vi "CSM Batch Format Tool.vi"() -> ()   [LabVIEW 2017]
uses:
  _csmHelper/Utility/CSM Module Type.ctl
  <vilib>/Utility/miscctls.llb/LVRectTypeDef.ctl
  _csmHelper/API/Destroy.vi
  _csmHelper/API/Save Instrument.vi
  _csmHelper/API/Create From Basic Refs.vi
  _csmHelper/Utility/Is CSM Module - VIRef.vi
  _Shared/CSM Shared.lvlib
  _csmDoc/csmdoc.lvlib
  Communicable State Machine.lvlib
  _csmHelper/Utility/CSM-Helper Utility.lvlib
  _csmHelper/CSM-Helper.lvclass
  _csmHelper/API/Open Front Panel.vi
panel:
  in  "Enum":enum16{"Debugging", "AutoErrorHandling"}(ring)
  in  "Option":bool
  in  "Open":bool
  in  "CSM Only?":bool
  in  "Terminate":bool
  in  "Refresh":bool
  in  "Action: Update Connect Panel Doc":bool
  in  "Action: Set Debugging":bool
  in  "Macro: Open If Inline":bool
  in  "Macro: Update VI Title":bool
  in  "Macro: Relocate VI Window":bool
  in  "Macro: Rename Year of copyright":bool
  out "Listbox":i32(listbox)
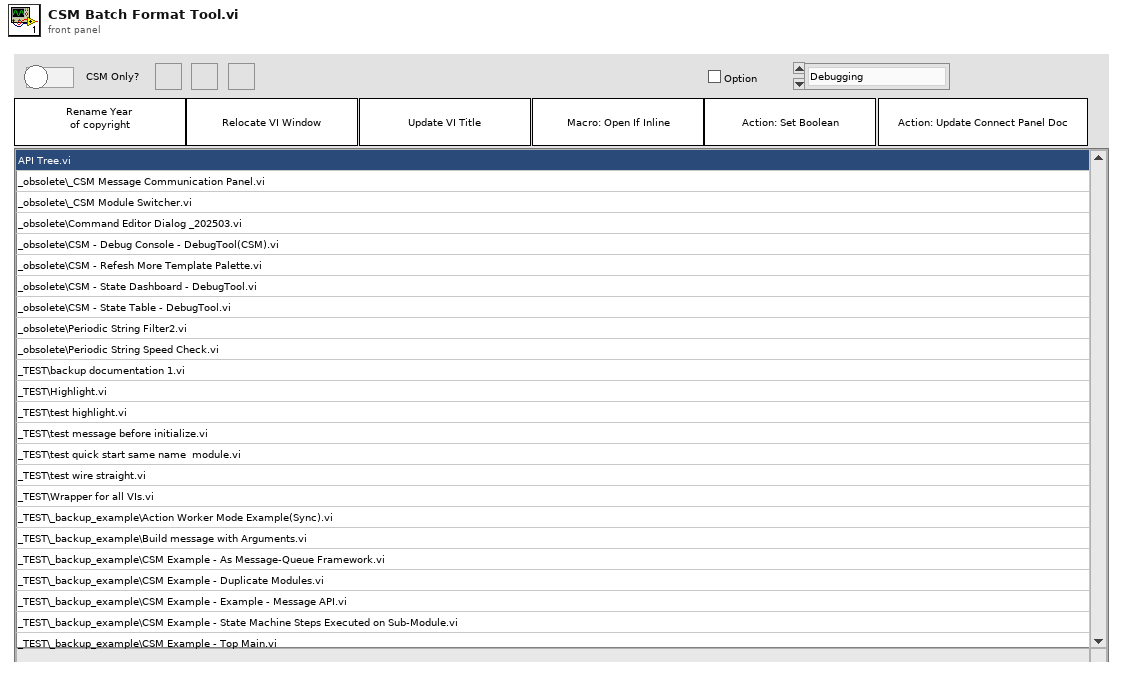
[diagram p1: front panel]
types:
  T1 = enum32{"Invalid", "Standard", "Closed", "Hidden", "Minimized", "Maximized"}
  T2 = enum32{"invalid app kind", "Development System", "Run Time System", "Student Edition", "Embedded LabVIEW", "Evaluation", "Custom"}
  T3 = typedef "CSM-Helper Utility.lvlib/CSM Module Type.ctl" = enum16{"Not a CSM", "JKISM", "CSM"}
  T4 = cluster{"Core":cluster{"Current VI Reference":refnum<vi>, "Close Panel on Exit?":bool}, "VIs":path[], "Success":bool, "Root":path}
  T5 = cluster{"Current VI Reference":refnum<vi>, "Close Panel on Exit?":bool}
  T6 = typedef "CSM-Helper Utility.lvlib/CSM Basic Refs.ctl" = cluster{"VI":refnum<vi>, "While Loop":refnum<vi>, "Case Structure":refnum<vi>, "Parse State Queue":refnum<vi>, "Event Structure":refnum<vi>, "Type":T3, "InLvlibp":bool}
  T7 = typedef "LVRectTypeDef.ctl" = cluster{"Left":i16, "Top":i16, "Right":i16, "Bottom":i16}
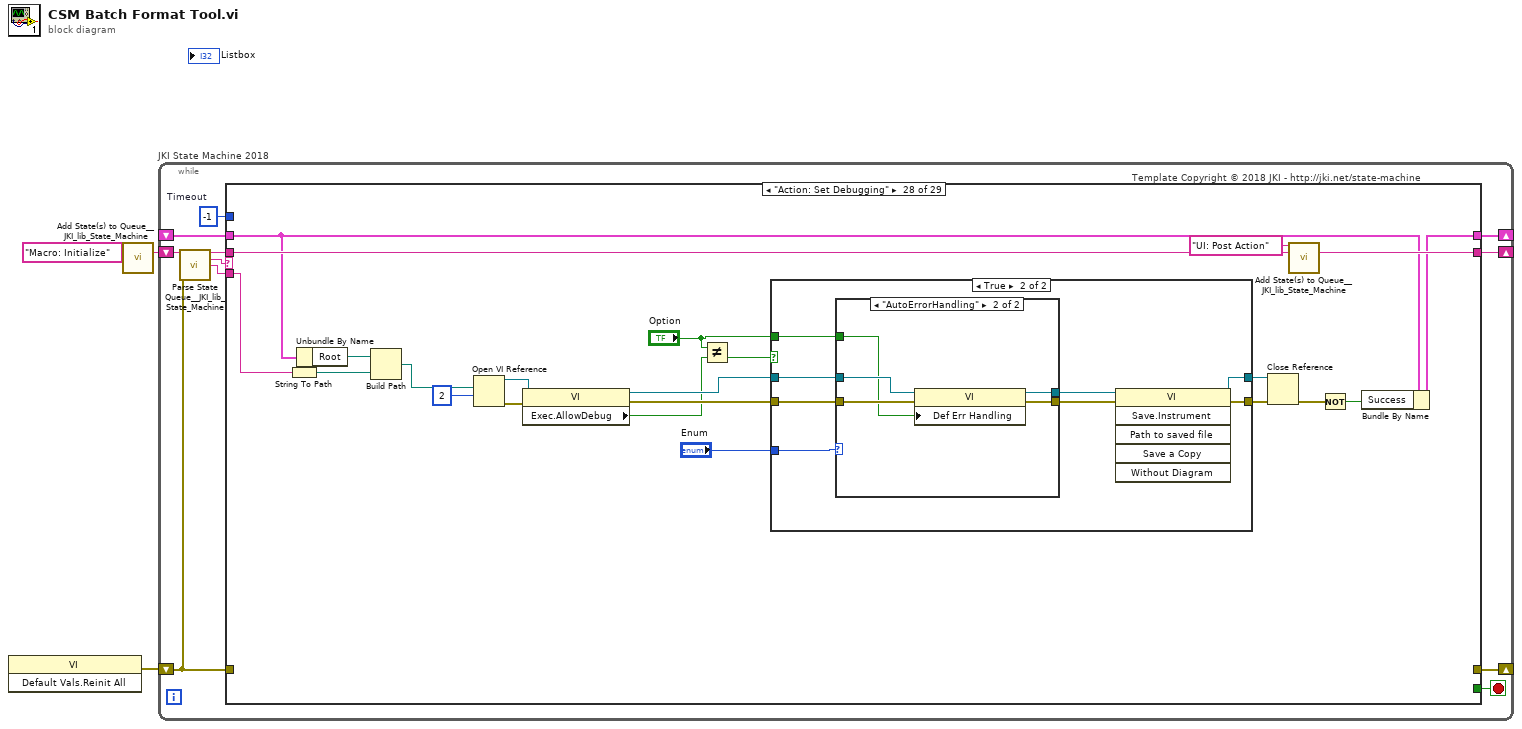
[diagram p0: block diagram]
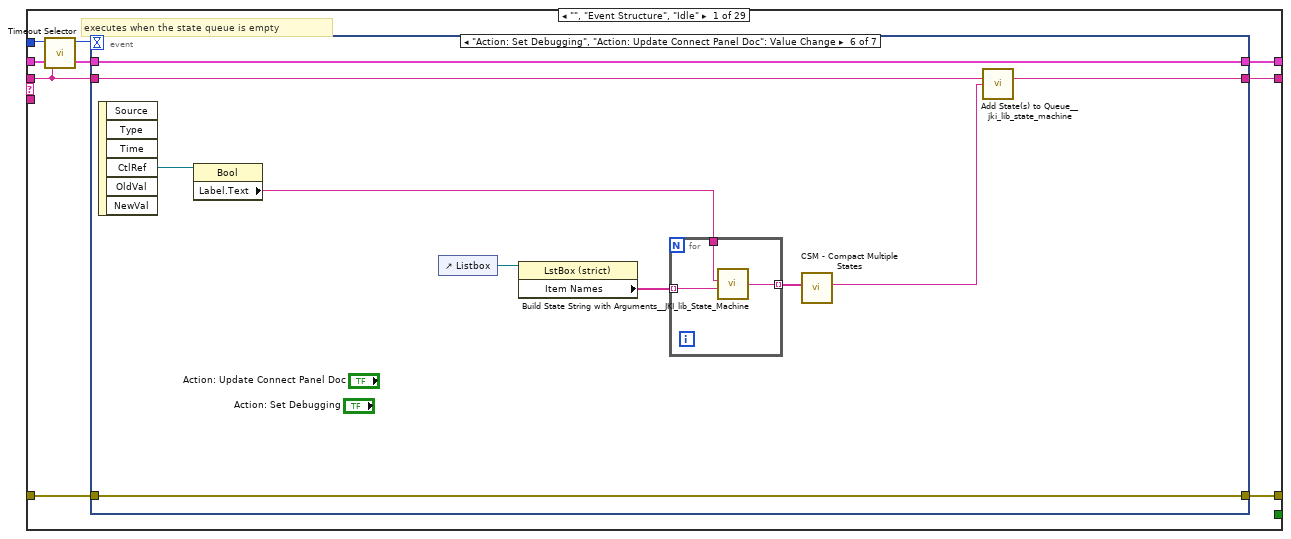
[diagram p2: hidden frame]
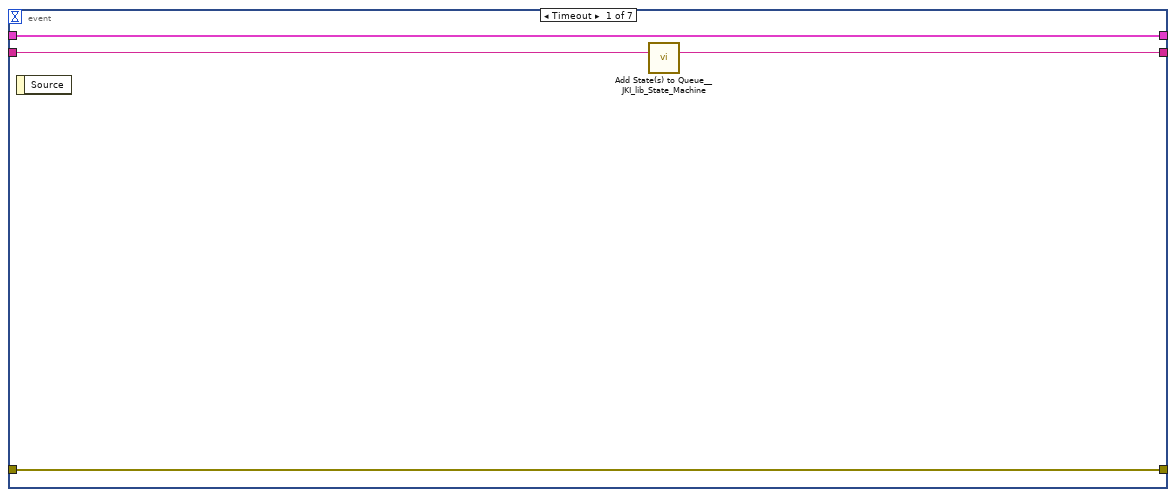
[diagram p3: hidden frame]
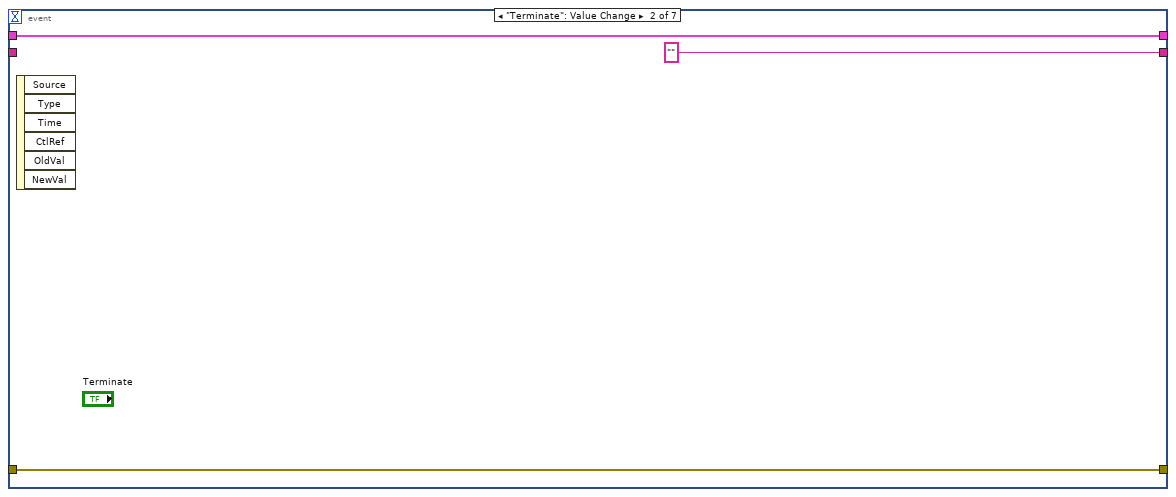
[diagram p4: hidden frame]
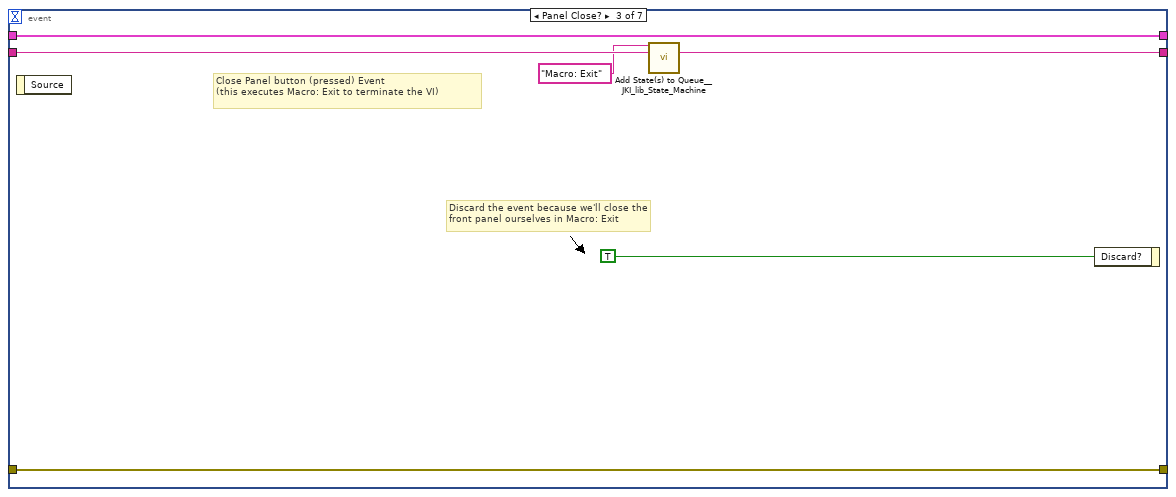
[diagram p5: hidden frame]
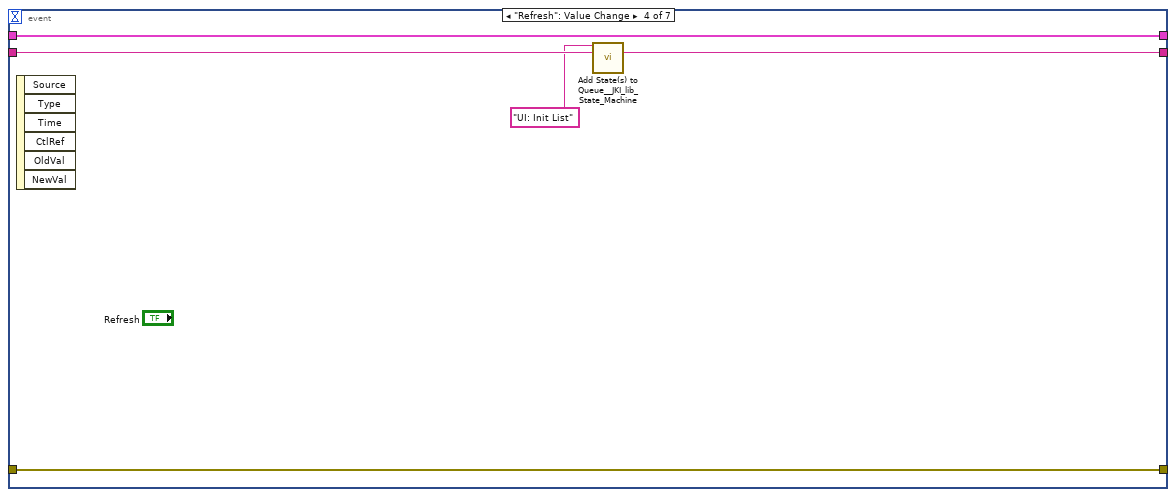
[diagram p6: hidden frame]
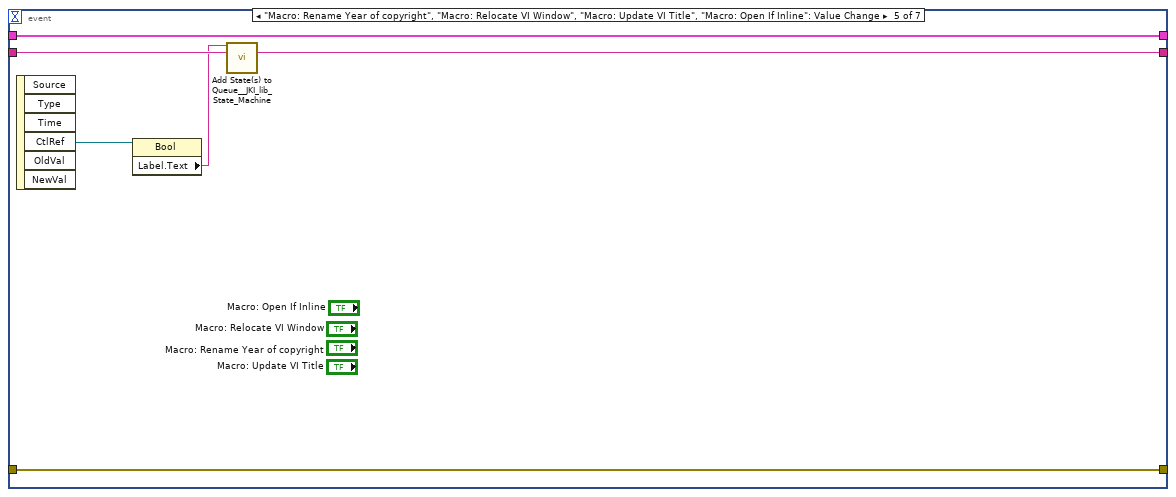
[diagram p7: hidden frame]
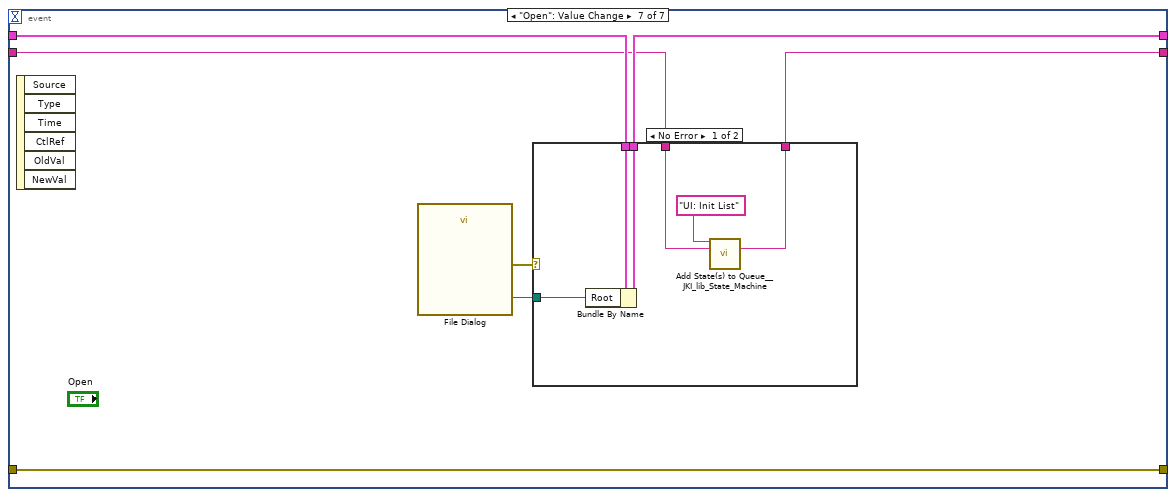
[diagram p8: hidden frame]
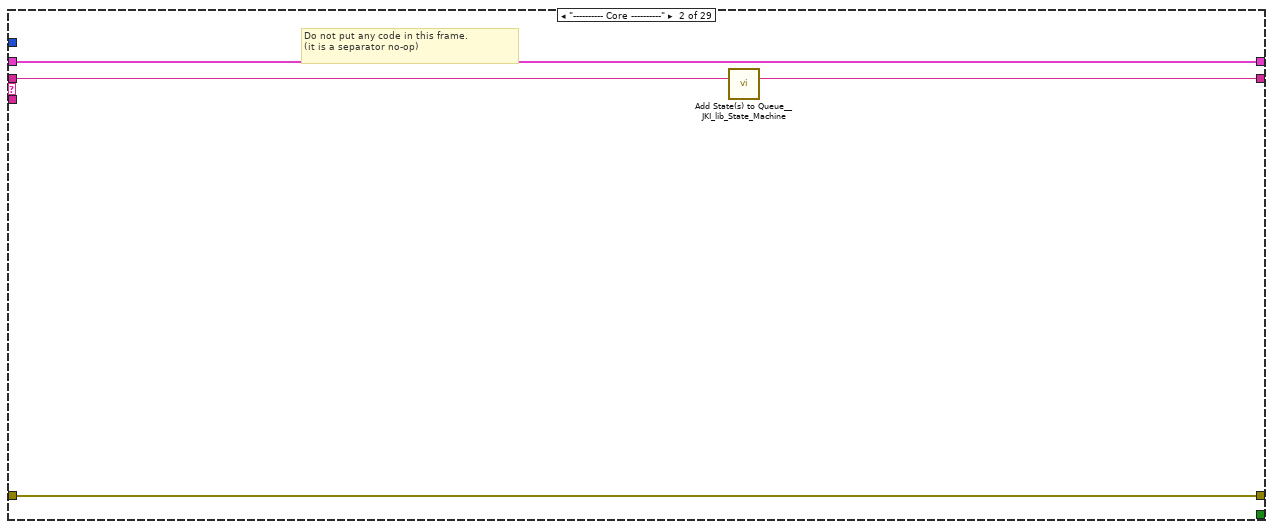
[diagram p10: hidden frame]
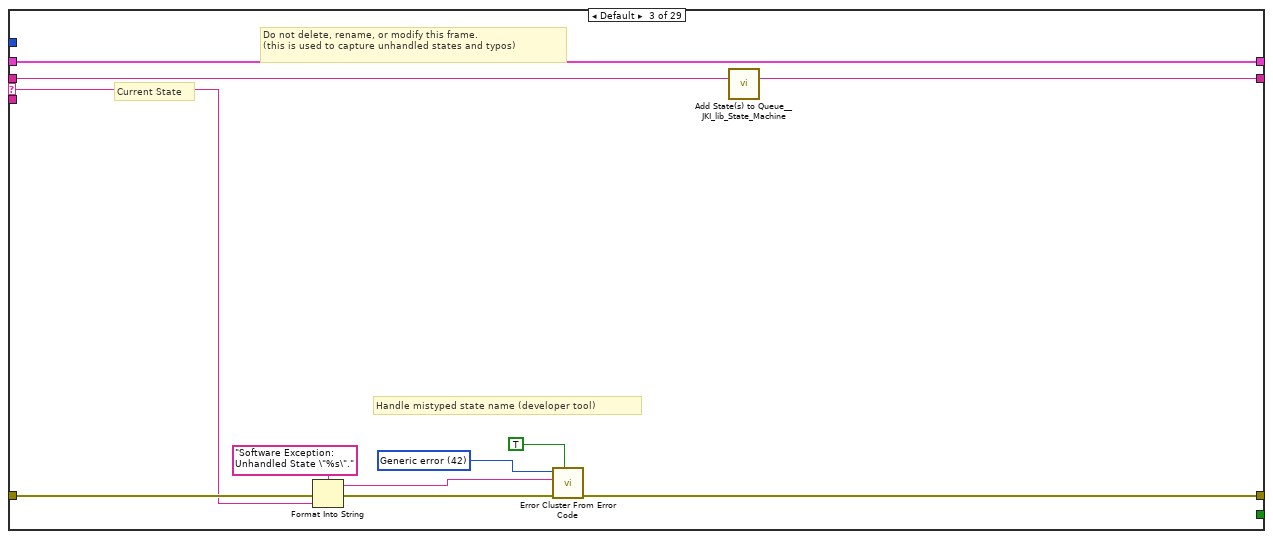
[diagram p11: hidden frame]
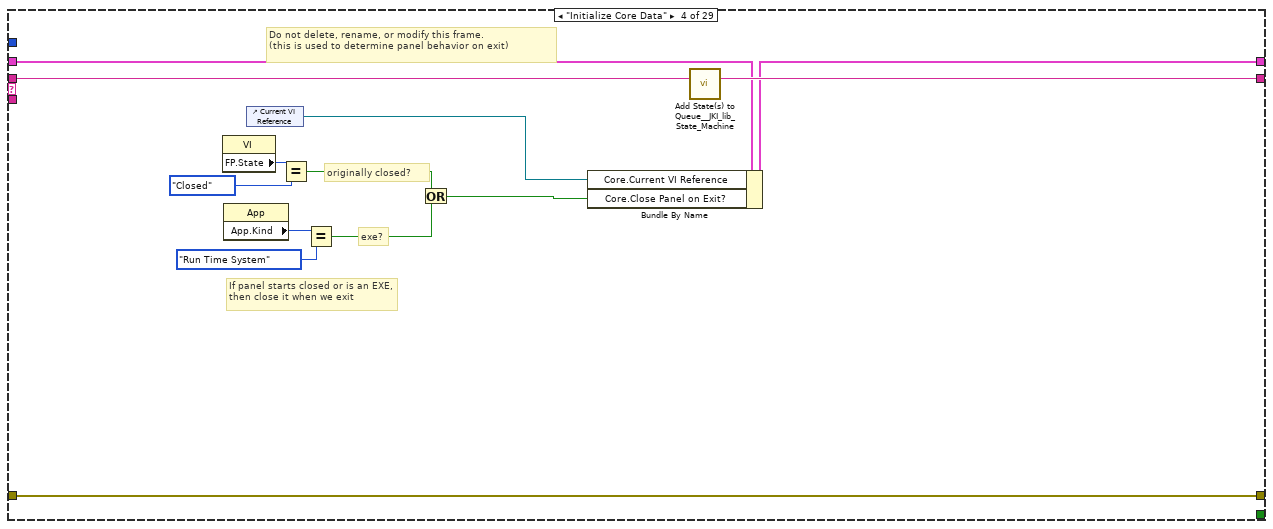
[diagram p12: hidden frame]
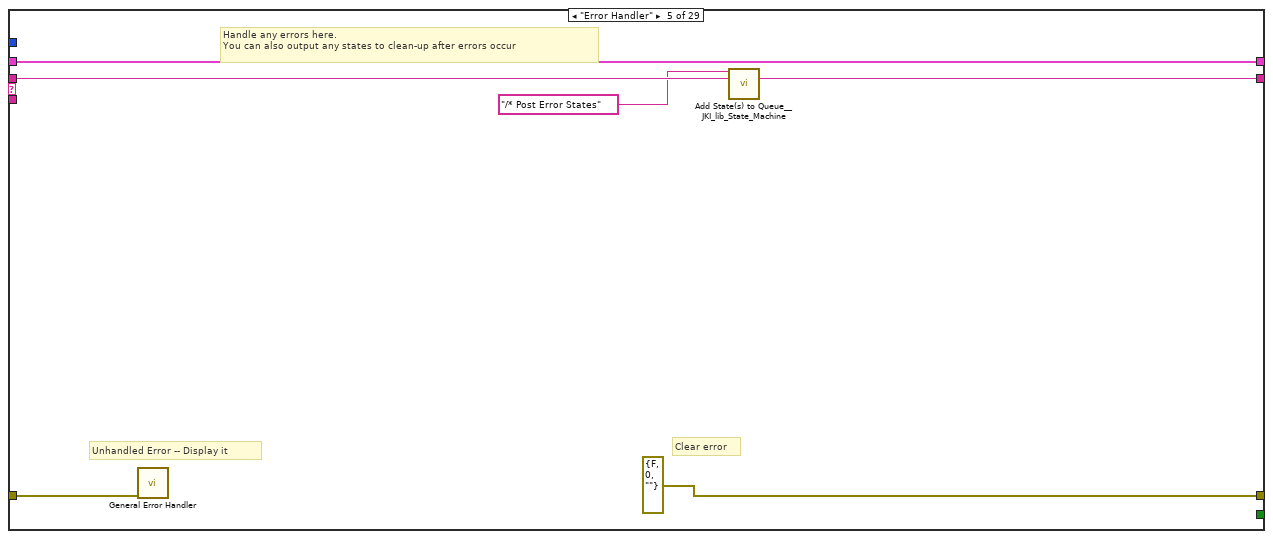
[diagram p13: hidden frame]
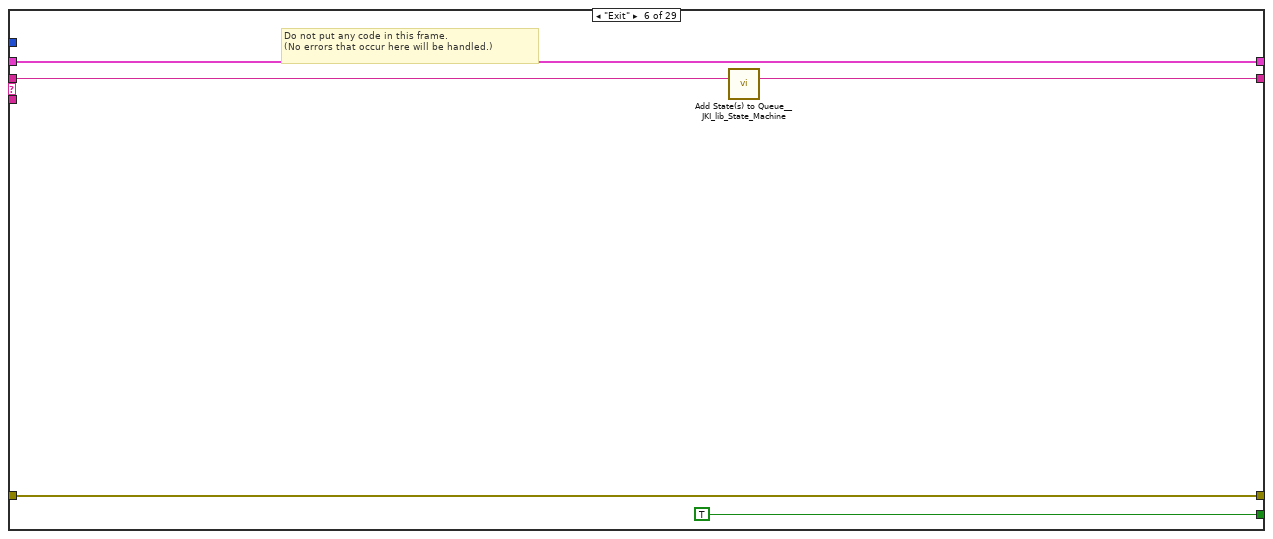
[diagram p14: hidden frame]
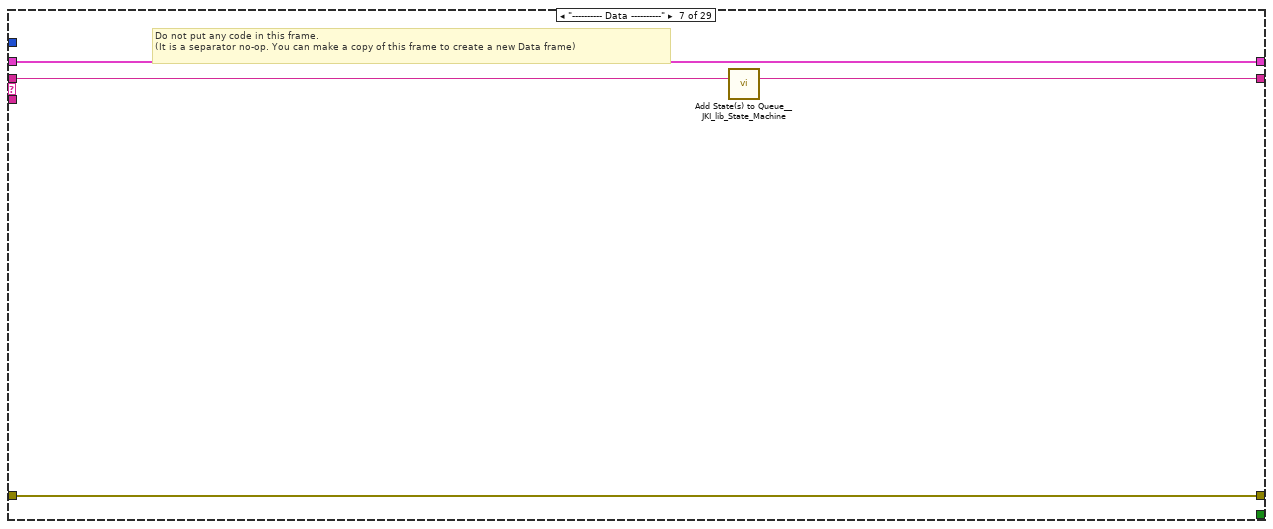
[diagram p15: hidden frame]
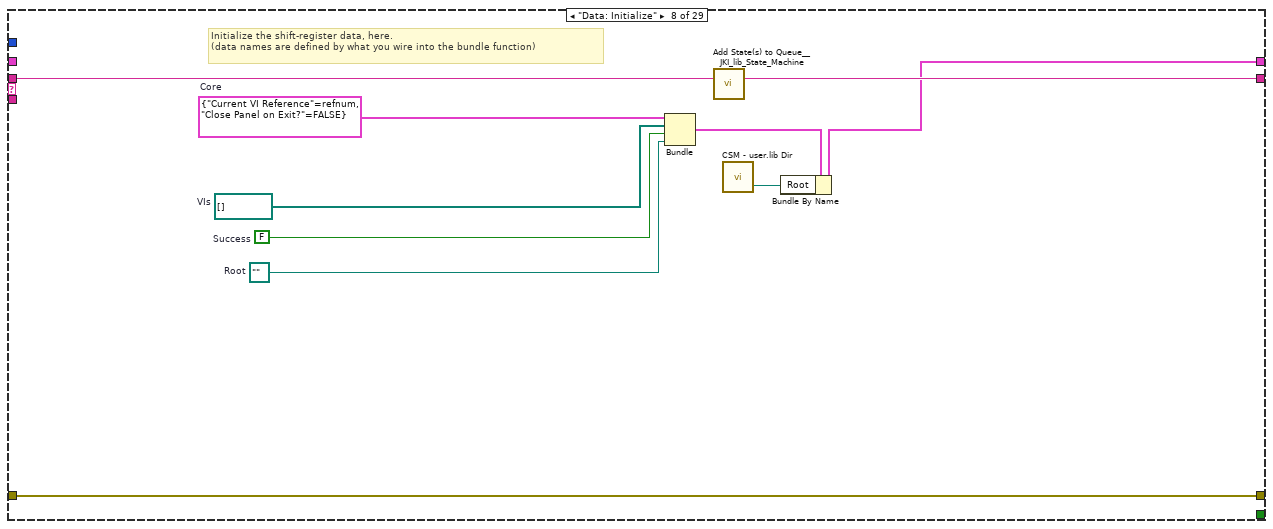
[diagram p16: hidden frame]
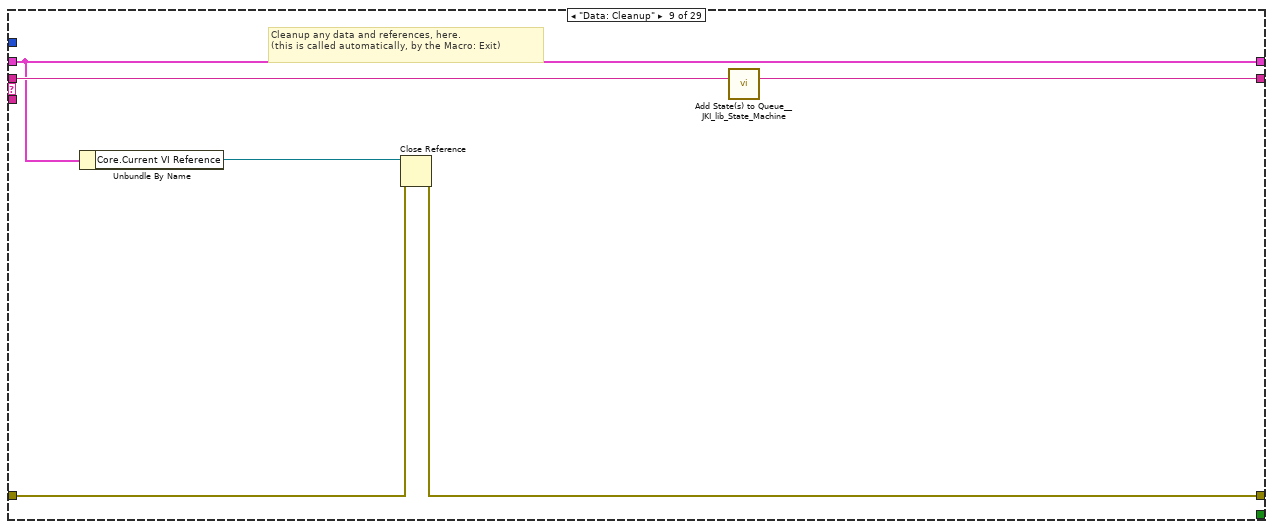
[diagram p17: hidden frame]
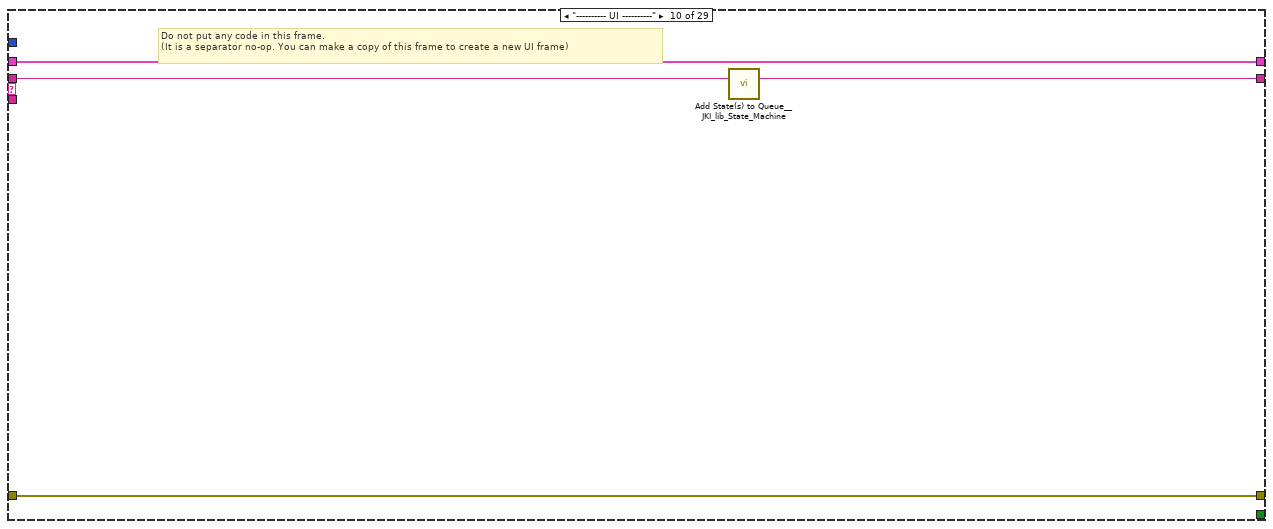
[diagram p18: hidden frame]
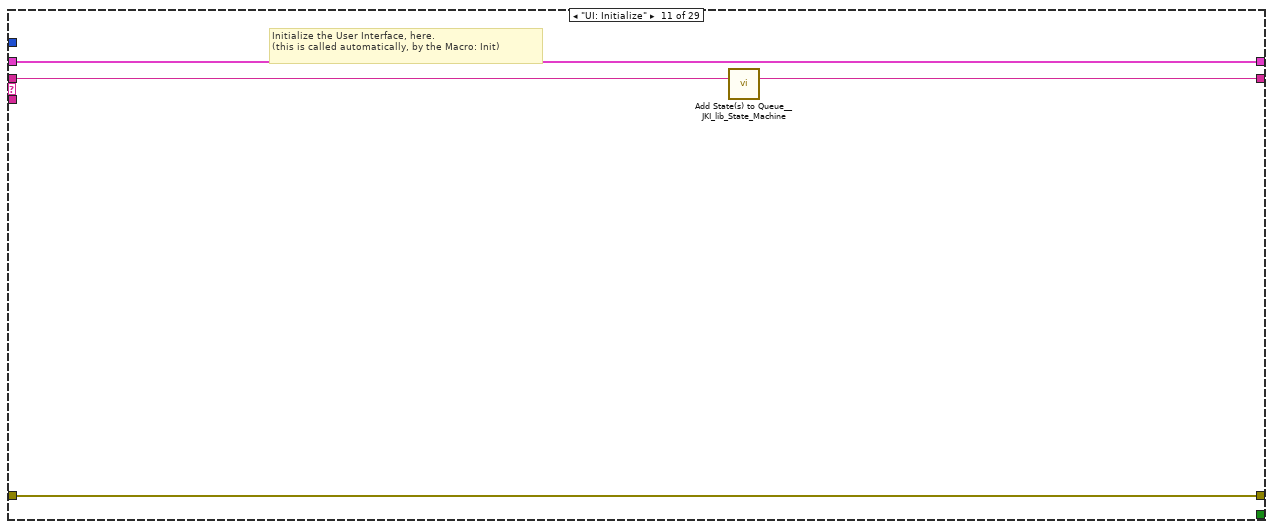
[diagram p19: hidden frame]
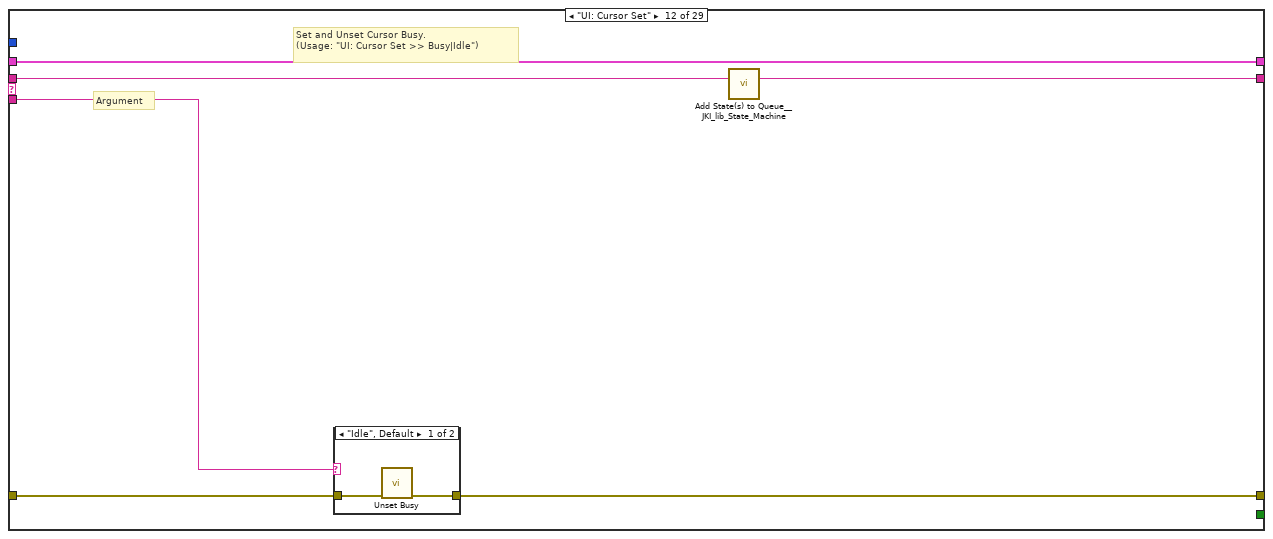
[diagram p20: hidden frame]
diagram:
  n1 = invoke class="VI" method="Default Vals.Reinit All"() -> (error out=w1:errorcluster)  [unwired: 3 in, 2 out]
  n2 = call <vilib>:"Add State(s) to Queue__JKI_lib_State_Machine.vi"("State(s) in (\"\")"="Macro: Initialize") -> ("States Out"=w3:string)  [unwired: 14 in]
  n3 = while "JKI State Machine 2018" {
    shift-right: [w7] -> _
    shift-left: _ -> [w6]
    shift-right: [w10] -> _
    shift-left: w1 -> [w4]
    shift-right: [w9] -> _
    shift-left: w3 -> [w11]
    stop <- w8 stop-if-true
    w5 = -1  # Timeout
    # "Template Copyright © 2018 JKI - http://jki.net/state-machine"
    n4 = call <vilib>:"Parse State Queue__JKI_lib_State_Machine.vi"("State Queue"=w11, "Error In (no error)"=w4) -> ("Remaining States"=w13:string, "Current State"=w14:string, "Arguments"=w12:string)  [unwired: 11 in]
    n5 = case shown="\"Action: Set Debugging\"" w14 {
      selector: w14 -> [_ _ w79 _ _ _ _ _ _ _ _ _ _ _ _ _ _ _ _ _ _ _ _ _ _ _ _ _ _]
      tunnel: w13 -> [w17 w78 w83 w102 w108 w113 w117 w127 w133 w137 w141 w147 w158 w238 w264 w288 w293 w303 w307 w315 w326 w337 w348 w356 w428 w475 w505 w547 w584]
      tunnel: w12 -> [_ _ _ _ _ _ _ _ _ _ _ w142 w152 _ _ _ _ _ _ _ _ _ _ w364 w433 w480 w502 w544 w581]
      tunnel: w6 -> [w21 w75 w81 w95 w105 w111 w114 _ w128 w134 w138 w145 w154 w226 w270 w285 w290 w300 w304 w312 w323 w334 w345 w352 w398 w469 w495 w537 w577]
      tunnel: [w20 w76 w85 w99 errorcluster {"status"=FALSE, "code"=0, "source"=""} ("error out") w110 w115 w124 w129 w135 w139 w143 w155 w239 w284 w286 w291 w301 w305 w313 w324 w335 w346 _ _ _ _ _ _] -> w10
      tunnel: w4 -> [w19 w76 w84 w99 w104 w110 w115 w124 w130 w135 w139 w144 w156 w239 w284 w286 w291 w301 w305 w313 w324 w335 w346 _ _ _ _ _ _]
      tunnel: [w22 w77 w82 w101 w107 w112 w116 w126 w132 w136 w140 w146 w157 w238 w265 w287 w292 w302 w306 w314 w325 w336 w347 w357 w429 w476 w506 w548 w585] -> w9
      tunnel: [_ _ _ _ _ TRUE _ _ _ _ _ _ _ _ _ _ _ _ _ _ _ _ _ _ _ _ _ _ _] -> w8
      tunnel: [w18 w75 w81 w100 w105 w111 w114 w119 w128 w134 w138 w145 w154 w228 w272 w285 w290 w300 w304 w312 w323 w334 w345 w360 w432 w479 w499 w541 w580] -> w7
      tunnel: w5 -> [w16 _ _ _ _ _ _ _ _ _ _ _ _ _ _ _ _ _ _ _ _ _ _ _ _ _ _ _ _]
      frame "", "Event Structure", "Idle" {
        # "executes when the state queue is empty"
        n6 = call "Timeout Selector.vi"("Remaining States"=w17, "Timeout Expected"=w16) -> ("Timeout"=w15:i32)  [unwired: 5 in]
        n7 = event shown="[5] \"Action: Set Debugging\", \"Action: Update Connect Panel Doc\": Value Change" {
          selector: _ -> [_ _ _ _ _ _ _]
          dyn-events: _ -> [_ _ _ _ _ _ _]
          timeout: w15 -> [_ _ _ _ _ _ _]
          tunnel: w17 -> [w26 _ w35 w37 w43 w51 w61]
          tunnel: [w25 "" ("States Out") w34 w38 w44 w52 w62] -> w22
          tunnel: w21 -> [w23 w28 w32 w39 w45 w55 w65]
          tunnel: [w24 w29 w33 w40 w46 w56 w66] -> w20
          tunnel: w19 -> [w24 w29 w33 w40 w46 w56 w66]
          tunnel: [w23 w28 w32 w39 w45 w55 w64] -> w18
          event Timeout {
            n8 = event-data() -> ()  [unwired: 1 in, 1 out]
            n9 = call <vilib>:"Add State(s) to Queue__JKI_lib_State_Machine.vi"("State(s) in (\"\")"=w26) -> ("States Out"=w25:string)  [unwired: 14 in]
          }
          event "Terminate": Value Change {
            n10 = event-data() -> ()  [unwired: 1 in, 6 out]
          }
          event Panel Close? {
            # "Discard the event because we'll close the front panel ourselves in Macro: Exit"
            # "Close Panel button (pressed) Event\n(this executes Macro: Exit to terminate the VI)"
            n11 = event-data() -> ()  [unwired: 1 in, 1 out]
            n12 = call <vilib>:"Add State(s) to Queue__JKI_lib_State_Machine.vi"("State(s) in Front (\"\")"="Macro: Exit", "State(s) in (\"\")"=w35) -> ("States Out"=w34:string)  [unwired: 13 in]
            n13 = event-data("Discard?"=TRUE) -> ()  [unwired: 1 in, 1 out]
          }
          event "Refresh": Value Change {
            n14 = event-data() -> ()  [unwired: 1 in, 6 out]
            n15 = call <vilib>:"Add State(s) to Queue__JKI_lib_State_Machine.vi"("State(s) in Front (\"\")"="UI: Init List" ("State(s) in Front (\"\")"), "State(s) in (\"\")"=w37) -> ("States Out"=w38:string)  [unwired: 13 in]
          }
          event "Macro: Rename Year of copyright", "Macro: Relocate VI Window", "Macro: Update VI Title", "Macro: Open If Inline": Value Change {
            n16 = event-data() -> ("CtlRef"=w42:refnum<vi>)  [unwired: 1 in, 5 out]
            n17 = property class="Bool"(reference=w42) -> ("Label.Text"=w41:string)  [unwired: 1 in, 2 out]
            n18 = call <vilib>:"Add State(s) to Queue__JKI_lib_State_Machine.vi"("State(s) in Front (\"\")"=w41, "State(s) in (\"\")"=w43) -> ("States Out"=w44:string)  [unwired: 13 in]
          }
          event "Action: Set Debugging", "Action: Update Connect Panel Doc": Value Change {
            n19 = event-data() -> ("CtlRef"=w49:refnum<vi>)  [unwired: 1 in, 5 out]
            n20 = property class="Bool"(reference=w49) -> ("Label.Text"=w48:string)  [unwired: 1 in, 2 out]
            n21 = control-ref of="Listbox"() -> (w47:refnum<vi>)
            n22 = property on="Property Node" class="LstBox (strict)"(reference=w47) -> ("Item Names"=w53:string[])  [unwired: 1 in, 2 out]
            n23 = for {
              tunnel: w53 -> [w59] mode=indexing
              tunnel: w48 -> [w58]
              tunnel: [w57] -> w54 mode=indexing
              n24 = call <vilib>:"Build State String with Arguments__JKI_lib_State_Machine.vi"("Arguments (\"\")"=w59, "State"=w58) -> ("State with Arguments"=w57:string)  [unwired: 4 in]
            }
            n25 = call "CSM - Compact Multiple States.vi"("Multiple States"=w54) -> ("States"=w50:string)  [unwired: 9 in]
            n26 = call <vilib>:"Add State(s) to Queue__jki_lib_state_machine.vi"("State(s) in (\"\")"=w51, "State(s) at Back (\"\")"=w50) -> ("States Out"=w52:string)  [unwired: 13 in]
          }
          event "Open": Value Change {
            n27 = event-data() -> ()  [unwired: 1 in, 6 out]
            n28 = call "File Dialog"() -> ("selected path"=w63:path, "error out"=w60:errorcluster)  [unwired: 12 in, 2 out]
            n29 = case shown="No Error" w60 {
              tunnel: w65 -> [w72 w74]
              tunnel: [w71 w74] -> w64
              tunnel: w63 -> [w70 _]
              tunnel: [w69 w73] -> w62
              tunnel: w61 -> [w68 w73]
              frame No Error {
                n30 = Bundle By Name(cluster=w72, "Root"=w70) -> (w71:T4)
                n31 = call <vilib>:"Add State(s) to Queue__JKI_lib_State_Machine.vi"("State(s) in Front (\"\")"="UI: Init List" ("State(s) in Front (\"\")"), "State(s) in (\"\")"=w68) -> ("States Out"=w69:string)  [unwired: 13 in]
              }
              frame Error {
              }
            }
          }
        }
      }
      frame "---------- Core ----------" {
        # "Do not put any code in this frame.\n(it is a separator no-op)"
        n32 = call <vilib>:"Add State(s) to Queue__JKI_lib_State_Machine.vi"("State(s) in (\"\")"=w78) -> ("States Out"=w77:string)  [unwired: 14 in]
      }
      frame Default {
        w88 = 42 items=["No error", "Argument error", "Memory is full", "Out of zone", "End of file", "File already open", "Generic file I/O error", "File not found", "File permission error", "Disk is full", "Duplicate path", "Too many files open", "System feature not enabled", "Resource file not found", "Cannot add resource", "Resource not found", "Image not found", "Image memory error", "Pen does not exist", "Config type invalid", "Config token not found", "Config parse error", "Config memory error", "Bad external code format", "Bad external code offset", "External code not present", "Null window", "Destroy window error", "Null menu", "Print aborted", "Bad print record", "Print driver error", "Windows error during printing", "Memory error during printing", "Print dialog error", "Generic print error", "Invalid device refnum", "Device not found", "Device parameter error", "Device unit error", "Cannot open device", "Device call aborted", "Generic error", "Cancelled by user", "Object ID too low", "Object ID too high", "Object not in heap", "Unknown heap", "Unknown object (invalid DefProc)", "Unknown object (DefProc not in table)", "Message out of range", "Invalid (null) method", "Unknown message", "Manager call not supported", "Bad address", "Network operation in progress", "Network operation timed out", "Connection is busy", "Network attribute not supported", "Network error", "Address in use", "System out of memory", "Connection aborted", "Connection refused", "Not connected", "Already connected", "Connection closed", "Initialization error (interapplication manager)", "Bad occurrence", "Wait on unbound occurrence handler", "Occurrence queue overflow", "Datalog type conflict", "Unused", "Unrecognized type (interapplication manager)", "Memory corrupt", "Failed to make temporary DLL", "Old CIN version", "Drag socket not found", "Failed to load drop-object", "Failed to register OLE object", "Failed to release OLE object", "Format specifier type mismatch", "Unknown format specifier", "Too few format specifiers", "Too many format specifiers", "Scan failed", "Newer CIN version", "Error converting to variant", "Runtime menu error", "Password tampered", "Variant attribute not found", "Incompatible variant data type", "Event data is not available", "Event Store is not present", "Occurrence is not found", "Event Queue is not created", "Event info is not available", "Refnum passed is NULL", "Error retrieving Class GUID", "Error retrieving CoClass GUID", "Error retrieving TypeLib GUID.", "Bad built application magic bytes.", "Specific driver is different from the specific driver associated with the Logical Name.", "There is no session opened to the class driver.", "Max Error", "MAX - Error with config objects", "MAX - Error loading configuration", "MAX - Group not supported"]
        # "Current State"
        # "Do not delete, rename, or modify this frame.\n(this is used to capture unhandled states and typos)"
        # "Handle mistyped state name (developer tool)"
        n33 = Format Into String(format string="Software Exception: Unhandled State \"%s\"." ("message"), error in=w84, w79) -> (resulting string=w87:string, error out=w86:errorcluster)  [unwired: 1 in]
        n34 = call <vilib>:"Error Cluster From Error Code.vi"("show call chain? (False)"=TRUE, "error in (no error)"=w86, "error message (\"\")"=w87, "error code (0)"=w88) -> ("error out"=w85:errorcluster)  [unwired: 5 in]
        n35 = call <vilib>:"Add State(s) to Queue__JKI_lib_State_Machine.vi"("State(s) in (\"\")"=w83) -> ("States Out"=w82:string)  [unwired: 14 in]
      }
      frame "Initialize Core Data" {
        # "Do not delete, rename, or modify this frame.\n(this is used to determine panel behavior on exit)"
        # "originally closed?"
        # "exe?"
        # "If panel starts closed or is an EXE, then close it when we exit"
        n36 = property class="VI"() -> ("FP.State"=w92:T1)  [unwired: 2 in, 2 out]
        n37 = property class="App"() -> ("App.Kind"=w98:T2)  [unwired: 2 in, 2 out]
        n38 = control-ref of="Current VI Reference"() -> (w93:refnum<vi>)
        n39 = Equal?(x=w92, y=T1."Closed" ("Front Panel Window:State")) -> (x = y?=w90:bool)
        n40 = Equal?(x=w98, y=T2."Run Time System" ("Application:Kind")) -> (x = y?=w96:bool)
        n41 = Or(x=w90, y=w96) -> (x .or. y?=w94:bool)
        n42 = Bundle By Name(cluster=w95, "Core.Current VI Reference"=w93, "Core.Close Panel on Exit?"=w94) -> (w100:T4)
        n43 = call <vilib>:"Add State(s) to Queue__JKI_lib_State_Machine.vi"("State(s) in (\"\")"=w102) -> ("States Out"=w101:string)  [unwired: 14 in]
      }
      frame "Error Handler" {
        # "Unhandled Error -- Display it"
        # "Handle any errors here.\nYou can also output any states to clean-up after errors occur"
        # "Clear error"
        n44 = call <vilib>:"General Error Handler.vi"("error in (no error)"=w104) -> ()  [unwired: 10 in, 5 out]
        n45 = call <vilib>:"Add State(s) to Queue__JKI_lib_State_Machine.vi"("State(s) in Front (\"\")"="/* Post Error States", "State(s) in (\"\")"=w108) -> ("States Out"=w107:string)  [unwired: 13 in]
      }
      frame "Exit" {
        # "Do not put any code in this frame.\n(No errors that occur here will be handled.)"
        n46 = call <vilib>:"Add State(s) to Queue__JKI_lib_State_Machine.vi"("State(s) in (\"\")"=w113) -> ("States Out"=w112:string)  [unwired: 14 in]
      }
      frame "---------- Data ----------" {
        # "Do not put any code in this frame.\n(It is a separator no-op. You can make a copy of this frame to create a new Data frame)"
        n47 = call <vilib>:"Add State(s) to Queue__JKI_lib_State_Machine.vi"("State(s) in (\"\")"=w117) -> ("States Out"=w116:string)  [unwired: 14 in]
      }
      frame "Data: Initialize" {
        w120 = path ""  # Root
        w121 = FALSE  # Success
        w122 = path[] []  # VIs
        w123 = T5 {"Current VI Reference"=refnum, "Close Panel on Exit?"=FALSE}  # Core
        # "Initialize the shift-register data, here.\n(data names are defined by what you wire into the bundle function)"
        n48 = Bundle("Core"=w123, "VIs"=w122, "Success"=w121, "Root"=w120) -> (w125:T4)  [unwired: 1 in]
        n49 = call <vilib>:"Add State(s) to Queue__JKI_lib_State_Machine.vi"("State(s) in (\"\")"=w127) -> ("States Out"=w126:string)  [unwired: 14 in]
        n50 = call "CSM - user.lib Dir.vi"() -> ("<LabVIEW>"=w118:path)  [unwired: 2 in, 1 out]
        n51 = Bundle By Name(cluster=w125, "Root"=w118) -> (w119:T4)
      }
      frame "Data: Cleanup" {
        # "Cleanup any data and references, here.\n(this is called automatically, by the Macro: Exit)"
        n52 = Unbundle By Name(w128) -> ("Core.Current VI Reference"=w131:refnum<vi>)
        n53 = Close Reference(reference=w131, error in (no error)=w130) -> (error out=w129:errorcluster)
        n54 = call <vilib>:"Add State(s) to Queue__JKI_lib_State_Machine.vi"("State(s) in (\"\")"=w133) -> ("States Out"=w132:string)  [unwired: 14 in]
      }
      frame "---------- UI ----------" {
        # "Do not put any code in this frame.\n(It is a separator no-op. You can make a copy of this frame to create a new UI frame)"
        n55 = call <vilib>:"Add State(s) to Queue__JKI_lib_State_Machine.vi"("State(s) in (\"\")"=w137) -> ("States Out"=w136:string)  [unwired: 14 in]
      }
      frame "UI: Initialize" {
        # "Initialize the User Interface, here.\n(this is called automatically, by the Macro: Init)"
        n56 = call <vilib>:"Add State(s) to Queue__JKI_lib_State_Machine.vi"("State(s) in (\"\")"=w141) -> ("States Out"=w140:string)  [unwired: 14 in]
      }
      frame "UI: Cursor Set" {
        # "Argument"
        # "Set and Unset Cursor Busy.\n(Usage: \"UI: Cursor Set >> Busy|Idle\")"
        n57 = case shown="\"Idle\", Default" w142 {
          tunnel: w144 -> [w149 w151]
          tunnel: [w148 w150] -> w143
          frame "Idle", Default {
            n58 = call <vilib>:"Unset Busy.vi"("error in (no error)"=w149) -> ("error out"=w148:errorcluster)  [unwired: 10 in]
          }
          frame "Busy" {
            n59 = call <vilib>:"Set Busy.vi"("error in (no error)"=w151) -> ("error out"=w150:errorcluster)  [unwired: 9 in, 1 out]
          }
        }
        n60 = call <vilib>:"Add State(s) to Queue__JKI_lib_State_Machine.vi"("State(s) in (\"\")"=w147) -> ("States Out"=w146:string)  [unwired: 14 in]
      }
      frame "UI: Front Panel State" {
        # "Argument"
        # "Set Front Panel Open or Closed\n(Usage: \"UI: Front Panel State >> Open|Close\")"
        n61 = Unbundle By Name(w154) -> ("Core.Current VI Reference"=w153:refnum<vi>)
        n62 = case shown="\"Minimize\", \"Minimized\"" w152 {
          tunnel: w156 -> [w164 w179 w190 w203 w216]
          tunnel: [w166 w180 w192 w205 w218] -> w155
          tunnel: w153 -> [w165 w177 w191 w204 w217]
          frame "Open", "Standard", Default {
            w159 = T1."Standard" ("State")
            n63 = property class="VI"(reference=w165, error in=w164) -> (reference out=w162:refnum<vi>, error out=w163:errorcluster, "FP.State"=w161:T1)
            n64 = Not Equal?(x=w161, y=w159) -> (x != y?=w160:bool)
            n65 = case shown="True" w160 {
              tunnel: [w170 w172] -> w166
              tunnel: w163 -> [w169 w172]
              tunnel: w162 -> [w168 _]
              tunnel: w159 -> [w167 _]
              frame True {
                n66 = invoke class="VI" method="FP.Open"(reference=w168, error in=w169, "Activate"=TRUE, "State"=w167) -> (error out=w170:errorcluster)  [unwired: 1 in, 4 out]
              }
              frame False {
              }
            }
          }
          frame "Close", "Closed" {
            n67 = property class="VI"(reference=w177, error in=w179) -> (reference out=w176:refnum<vi>, error out=w178:errorcluster, "FP.State"=w174:T1)
            n68 = Not Equal?(x=w174, y=T1."Closed" ("Front Panel Window:State")) -> (x != y?=w173:bool)
            n69 = case shown="True" w173 {
              tunnel: [w181 w184] -> w180
              tunnel: w178 -> [w181 w183]
              tunnel: w176 -> [_ w182]
              frame False {
              }
              frame True {
                n70 = invoke class="VI" method="FP.Close"(reference=w182, error in=w183) -> (error out=w184:errorcluster)  [unwired: 1 in, 2 out]
              }
            }
          }
          frame "Hidden", "Hide" {
            w185 = T1."Hidden" ("State")
            n71 = property class="VI"(reference=w191, error in=w190) -> (reference out=w188:refnum<vi>, error out=w189:errorcluster, "FP.State"=w187:T1)
            n72 = Not Equal?(x=w187, y=w185) -> (x != y?=w186:bool)
            n73 = case shown="True" w186 {
              tunnel: [w196 w197] -> w192
              tunnel: w189 -> [w195 w197]
              tunnel: w188 -> [w194 _]
              tunnel: w185 -> [w193 _]
              frame True {
                n74 = invoke class="VI" method="FP.Open"(reference=w194, error in=w195, "State"=w193) -> (error out=w196:errorcluster)  [unwired: 2 in, 4 out]
              }
              frame False {
              }
            }
          }
          frame "Minimize", "Minimized" {
            w198 = T1."Minimized" ("State")
            n75 = property class="VI"(reference=w204, error in=w203) -> (reference out=w201:refnum<vi>, error out=w202:errorcluster, "FP.State"=w200:T1)
            n76 = Not Equal?(x=w200, y=w198) -> (x != y?=w199:bool)
            n77 = case shown="True" w199 {
              tunnel: [w209 w210] -> w205
              tunnel: w202 -> [w208 w210]
              tunnel: w201 -> [w207 _]
              tunnel: w198 -> [w206 _]
              frame True {
                n78 = invoke class="VI" method="FP.Open"(reference=w207, error in=w208, "State"=w206) -> (error out=w209:errorcluster)  [unwired: 2 in, 4 out]
              }
              frame False {
              }
            }
          }
          frame "Maximize", "Maximized" {
            w211 = T1."Maximized" ("State")
            n79 = property class="VI"(reference=w217, error in=w216) -> (reference out=w214:refnum<vi>, error out=w215:errorcluster, "FP.State"=w213:T1)
            n80 = Not Equal?(x=w213, y=w211) -> (x != y?=w212:bool)
            n81 = case shown="True" w212 {
              tunnel: [w222 w223] -> w218
              tunnel: w215 -> [w221 w223]
              tunnel: w214 -> [w220 _]
              tunnel: w211 -> [w219 _]
              frame True {
                n82 = invoke class="VI" method="FP.Open"(reference=w220, error in=w221, "State"=w219) -> (error out=w222:errorcluster)  [unwired: 2 in, 4 out]
              }
              frame False {
              }
            }
          }
        }
        n83 = call <vilib>:"Add State(s) to Queue__JKI_lib_State_Machine.vi"("State(s) in (\"\")"=w158) -> ("States Out"=w157:string)  [unwired: 14 in]
      }
      frame "UI: Init List" {
        w233 = 0 ("Top Row")
        n84 = Unbundle By Name(w226) -> ("Root"=w224:path)
        n85 = case shown="True" "CSM Only?" {
          tunnel: [w240 w247] -> w232
          tunnel: w224 -> [w241 _]
          frame False {
            n86 = for {
              tunnel: w241 -> [w245]
              tunnel: string[] ["*.vi", "*.vim", "*.vit"] -> [w244] mode=indexing
              tunnel: [w243] -> w240 mode=concatenating
              n87 = call <vilib>:"Recursive File List.vi"("pattern"=w244, "Folder Path"=w245) -> ("All Files in Dir"=w243:path[])  [unwired: 5 in, 4 out]
            }
          }
          frame True {
            n88 = call "_list_CSM documented VIs.vi"("Only CSM Folder"=FALSE) -> ("Array"=w248:path[])  [unwired: 10 in]
            n89 = for {
              tunnel: w248 -> [w254] mode=indexing
              tunnel: [w254] -> w247 mode=indexing if=w251
              n90 = Open VI Reference(vi path=w254, options=32) -> (vi reference=w253:refnum<vi>, error out=w255:errorcluster)  [unwired: 4 in]
              n91 = call-poly "Is CSM Module.vi"("error in (no error)"=w255, "VIRef"=w253) -> ("error out"=w256:errorcluster, "CSMType"=w250:T3)  [unwired: 6 in, 2 out]
              n92 = Close Reference(reference=w253, error in (no error)=w256) -> ()  [unwired: 1 out]
              n93 = Equal?(x=CSM_Module_Type."CSM", y=w250) -> (x = y?=w251:bool)
            }
          }
        }
        n94 = Path to Array of Strings(0:w224) -> (2:w231:string[])  [unwired: 1 out]
        n95 = Array Size(array=w231) -> (size(s)=w230:i32)
        n96 = Path To String(path=w224) -> (string=w225:string)
        n97 = for {
          tunnel: w232 -> [w262] mode=indexing
          tunnel: w230 -> [w260]
          tunnel: [w259] -> w229 mode=indexing
          n98 = Path to Array of Strings(0:w262) -> (2:w261:string[])  [unwired: 1 out]
          n99 = Array Subset(array=w261, index=w260) -> (w258:string[])  [unwired: 1 in]
          n100 = Array of Strings to Path(0:w258, 1:TRUE ("relative")) -> (2:w259:path)
        }
        n101 = property class="VI"("Front Panel.Title"=w225) -> ()  [unwired: 2 in, 2 out]
        n102 = Path To String(path=w229) -> (string=w236:string[])
        n103 = Array Size(array=w236) -> (size(s)=w237:i32)
        n104 = Bundle By Name(cluster=w226, "VIs"=w229) -> (w228:T4)
        n105 = Initialize Array(0 ("Top Row"), w237) -> (w234:i32[])
        n106 = property on="Listbox" class="LstBox (strict)"("Item Names"=w236, "Top Row"=w233, "Item Symbols"=w234, "Value"=w233) -> ()  [unwired: 2 in, 2 out]
      }
      frame "UI: Post Action" {
        n107 = Unbundle By Name(w270) -> ("Success"=w269:bool)
        n108 = control-ref of="Listbox"() -> (w275:refnum<vi>)
        n109 = property on="Property Node" class="LstBox (strict)"(reference=w275) -> (reference out=w274:refnum<vi>, error out=w273:errorcluster, "Value"=w276:i32, "Item Symbols"=w283:i32[])  [unwired: 1 in]
        n110 = Select(t=1 ("new element/subarray"), s=w269, f=2 ("new element/subarray")) -> (s? t:f=w266:i32)
        n111 = Replace Array Subset(array=w283, new element=w266, index=w276) -> (w282:i32[])
        n112 = Subtract(x=w276, y=5) -> (x-y=w279:i32)
        n113 = Increment(x=w276) -> (x+1=w281:i32)
        n114 = Max & Min(x=w279, y=0) -> (max(x,y)=w277:i32)  [unwired: 1 out]
        n115 = property on="Property Node" class="LstBox (strict)"(reference=w274, error in=w273, "Top Row"=w277, "Item Symbols"=w282, "Value"=w281) -> ()  [unwired: 2 out]
        n116 = Bundle By Name(cluster=w270, "Success"=TRUE ("Last Action Success")) -> (w272:T4)
        n117 = call <vilib>:"Add State(s) to Queue__JKI_lib_State_Machine.vi"("State(s) in Front (\"\")"="Idle" ("State(s) in Front (\"\")"), "State(s) in (\"\")"=w264) -> ("States Out"=w265:string)  [unwired: 13 in]
      }
      frame "---------- Macro ----------" {
        # "Do not put any code in this frame.\n(It is a separator no-op. You can make a copy of this frame to create a new Macro frame)"
        n118 = call <vilib>:"Add State(s) to Queue__JKI_lib_State_Machine.vi"("State(s) in (\"\")"=w288) -> ("States Out"=w287:string)  [unwired: 14 in]
      }
      frame "Macro: Initialize" {
        # "Initialization Macro\n(This is called once, when the VI starts)"
        n119 = call <vilib>:"Add State(s) to Queue__JKI_lib_State_Machine.vi"("State(s) in Front (\"\")"="Data: Initialize\nInitialize Core Data\nUI: Initialize\nUI: Front Panel State >> Open\nUI: Init List", "State(s) in (\"\")"=w293) -> ("States Out"=w292:string)  [unwired: 13 in]
      }
      frame "Macro: Exit" {
        # "Exit Macro\n(This is called once, when the VI exits)"
        n120 = Unbundle By Name(w300) -> ("Core.Close Panel on Exit?"=w299:bool)
        n121 = Select(t="UI: Front Panel State >> Close", s=w299, f="") -> (s? t:f=w296:string)
        n122 = call <vilib>:"Add State(s) to Queue__JKI_lib_State_Machine.vi"("State(s) in (\"\")"=w296, "State(s) at Back (\"\")"="Data: Cleanup\nExit") -> ("States Out"=w294:string)  [unwired: 13 in]
        n123 = call <vilib>:"Add State(s) to Queue__JKI_lib_State_Machine.vi"("State(s) in Front (\"\")"=w294, "State(s) in (\"\")"=w303) -> ("States Out"=w302:string)  [unwired: 13 in]
      }
      frame "---------- Action ----------" {
        # "Template Separator\n(You can make a copy of, or modify, this frame)"
        n124 = call <vilib>:"Add State(s) to Queue__JKI_lib_State_Machine.vi"("State(s) in (\"\")"=w307) -> ("States Out"=w306:string)  [unwired: 14 in]
      }
      frame "Macro: Rename Year of copyright" {
        n125 = property on="Listbox" class="LstBox (strict)"() -> ("Item Names"=w311:string[])  [unwired: 2 in, 2 out]
        n126 = for {
          tunnel: w311 -> [w318] mode=indexing
          tunnel: "Action: Rename Year of copyright" ("State") -> [w317]
          tunnel: [w316] -> w309 mode=indexing
          n127 = call <vilib>:"Build State String with Arguments__JKI_lib_State_Machine.vi"("Arguments (\"\")"=w318, "State"=w317) -> ("State with Arguments"=w316:string)  [unwired: 4 in]
        }
        n128 = call "CSM - Compact Multiple States.vi"("Multiple States"=w309) -> ("States"=w308:string)  [unwired: 9 in]
        n129 = call <vilib>:"Add State(s) to Queue__JKI_lib_State_Machine.vi"("State(s) in Front (\"\")"=w308, "State(s) in (\"\")"=w315) -> ("States Out"=w314:string)  [unwired: 13 in]
      }
      frame "Macro: Relocate VI Window" {
        n130 = property on="Listbox" class="LstBox (strict)"() -> ("Item Names"=w322:string[])  [unwired: 2 in, 2 out]
        n131 = for {
          tunnel: w322 -> [w329] mode=indexing
          tunnel: "Action: Relocate VI Window" ("State") -> [w328]
          tunnel: [w327] -> w320 mode=indexing
          n132 = call <vilib>:"Build State String with Arguments__JKI_lib_State_Machine.vi"("Arguments (\"\")"=w329, "State"=w328) -> ("State with Arguments"=w327:string)  [unwired: 4 in]
        }
        n133 = call "CSM - Compact Multiple States.vi"("Multiple States"=w320) -> ("States"=w319:string)  [unwired: 9 in]
        n134 = call <vilib>:"Add State(s) to Queue__JKI_lib_State_Machine.vi"("State(s) in Front (\"\")"=w319, "State(s) in (\"\")"=w326) -> ("States Out"=w325:string)  [unwired: 13 in]
      }
      frame "Macro: Update VI Title" {
        n135 = property on="Listbox" class="LstBox (strict)"() -> ("Item Names"=w333:string[])  [unwired: 2 in, 2 out]
        n136 = for {
          tunnel: w333 -> [w340] mode=indexing
          tunnel: "Action: Update VI Title" ("State") -> [w339]
          tunnel: [w338] -> w331 mode=indexing
          n137 = call <vilib>:"Build State String with Arguments__JKI_lib_State_Machine.vi"("Arguments (\"\")"=w340, "State"=w339) -> ("State with Arguments"=w338:string)  [unwired: 4 in]
        }
        n138 = call "CSM - Compact Multiple States.vi"("Multiple States"=w331) -> ("States"=w330:string)  [unwired: 9 in]
        n139 = call <vilib>:"Add State(s) to Queue__JKI_lib_State_Machine.vi"("State(s) in Front (\"\")"=w330, "State(s) in (\"\")"=w337) -> ("States Out"=w336:string)  [unwired: 13 in]
      }
      frame "Macro: Open If Inline" {
        n140 = property on="Listbox" class="LstBox (strict)"() -> ("Item Names"=w344:string[])  [unwired: 2 in, 2 out]
        n141 = for {
          tunnel: w344 -> [w351] mode=indexing
          tunnel: "Action: Open If Inline" ("State") -> [w350]
          tunnel: [w349] -> w342 mode=indexing
          n142 = call <vilib>:"Build State String with Arguments__JKI_lib_State_Machine.vi"("Arguments (\"\")"=w351, "State"=w350) -> ("State with Arguments"=w349:string)  [unwired: 4 in]
        }
        n143 = call "CSM - Compact Multiple States.vi"("Multiple States"=w342) -> ("States"=w341:string)  [unwired: 9 in]
        n144 = call <vilib>:"Add State(s) to Queue__JKI_lib_State_Machine.vi"("State(s) in Front (\"\")"=w341, "State(s) in (\"\")"=w348) -> ("States Out"=w347:string)  [unwired: 13 in]
      }
      frame "Action: Rename Year of copyright" {
        n145 = String To Path(string=w364) -> (path=w365:path)
        n146 = Unbundle By Name(w352) -> ("Root"=w353:path)
        n147 = Build Path(base path=w353, name or relative path=w365) -> (appended path=w363:path)
        n148 = call <vilib>:"Check if File or Folder Exists.vi"("path"=w363) -> ("error out"=w361:errorcluster, "file or folder exists?"=w354:bool, "dup path"=w362:path)  [unwired: 8 in]
        n149 = case shown="True" w354 {
          tunnel: w362 -> [_ w368]
          tunnel: w361 -> [w366 w369]
          tunnel: [w366 w367] -> w359
          frame False {
          }
          frame True {
            n150 = Open VI Reference(vi path=w368, options=2, error in (no error)=w369) -> (vi reference=w372:refnum<vi>, error out=w373:errorcluster)  [unwired: 3 in]
            n151 = call-poly "Is CSM Module.vi"("error in (no error)"=w373, "VIRef"=w372) -> ("error out"=w371:errorcluster, "Is CSM Module?"=w374:bool, "CSM Basic Refs"=w370:T6)  [unwired: 6 in, 1 out]
            n152 = case shown="True" w374 {
              tunnel: [w378 w391] -> w367
              tunnel: w370 -> [w377 w390]
              tunnel: w371 -> [w379 w389]
              frame False {
                n153 = Unbundle By Name(w377) -> ("VI"=w376:refnum<vi>)
                n154 = Close Reference(reference=w376, error in (no error)=w379) -> (error out=w378:errorcluster)
              }
              frame True {
                n155 = call-poly "CSM-Helper API.vi"("error in (no error)"=w389, "CSM Basic Refs"=w390) -> ("error out"=w386:errorcluster, "CSM-Helper.lvclass"=w387:refnum<class "CSM-Helper.lvclass">)  [unwired: 8 in]
                n156 = Get Date/Time In Seconds() -> (seconds since 1Jan1904=w388:timestamp)
                n157 = disable-structure shown="Disabled" {
                  disable-tunnel: w387 -> [w395 w396]
                  disable-tunnel: w386 -> [w394 w397]
                  disable-tunnel: [w393 w397] -> w385
                  disable-tunnel: [w392 w396] -> w384
                  frame Disabled {
                    n158 = call-poly "CSM-Helper API.vi"("error in (no error)"=w394, "CSM-Helper in"=w395) -> ("error out"=w393:errorcluster, "CSM-Helper out"=w392:refnum<class "CSM-Helper.lvclass">)  [unwired: 8 in]
                  }
                  frame Enabled {
                  }
                }
                n159 = call "Rename Copyright Year.vi"("error in (no error)"=w385, "seconds since 1Jan1904"=w388, "CSM-Helper in"=w384) -> ("error out"=w380:errorcluster, "CSM-Helper out"=w381:refnum<class "CSM-Helper.lvclass">)  [unwired: 7 in]
                n160 = call-poly "CSM-Helper API.vi"("error in (no error)"=w380, "CSM-Helper in"=w381) -> ("error out"=w382:errorcluster, "CSM-Helper out"=w383:refnum<class "CSM-Helper.lvclass">)  [unwired: 8 in]
                n161 = call-poly "CSM-Helper API.vi"("error in (no error)"=w382, "CSM-Helper in"=w383) -> ("error out"=w391:errorcluster)  [unwired: 8 in, 1 out]
              }
            }
          }
        }
        n162 = call <vilib>:"Add State(s) to Queue__JKI_lib_State_Machine.vi"("State(s) in Front (\"\")"="UI: Post Action" ("State(s) in Front (\"\")"), "State(s) in (\"\")"=w356) -> ("States Out"=w357:string)  [unwired: 13 in]
        n163 = Not(x=w359) -> (.not. x?=w358:bool)
        n164 = Bundle By Name(cluster=w352, "Success"=w358) -> (w360:T4)
      }
      frame "Action: Relocate VI Window" {
        w414 = T7 {"Left"=110, "Top"=110, "Right"=0, "Bottom"=0} ("Front Panel Window:Window Bounds")
        w413 = T7 {"Left"=100, "Top"=100, "Right"=0, "Bottom"=0} ("Front Panel Window:Window Bounds")
        n165 = String To Path(string=w433) -> (path=w434:path)
        n166 = Unbundle By Name(w398) -> ("Root"=w399:path)
        n167 = Build Path(base path=w399, name or relative path=w434) -> (appended path=w425:path)
        n168 = Open VI Reference(vi path=w425, options=2) -> (vi reference=w417:refnum<vi>, error out=w420:errorcluster)  [unwired: 4 in]
        n169 = disable-structure shown="Disabled" {
          disable-tunnel: w420 -> [w460 w462]
          disable-tunnel: [w459 w462] -> w419
          disable-tunnel: [w458 w461] -> w418
          disable-tunnel: w417 -> [w457 w461]
          frame Disabled {
            n170 = invoke class="VI" method="FP.Open"(reference=w457, error in=w460) -> (reference out=w458:refnum<vi>, error out=w459:errorcluster)  [unwired: 3 in, 3 out]
          }
          frame Enabled {
          }
        }
        n171 = property class="VI"(reference=w418, error in=w419) -> (reference out=w424:refnum<vi>, error out=w423:errorcluster, "Front Panel.WinBounds"=w416:T7, "BDWin.Bounds"=w415:T7)
        n172 = Unbundle(w413) -> ("Left"=w406:i16, "Top"=w407:i16)  [unwired: 2 out]
        n173 = Unbundle(w415) -> ("Left"=w412:i16, "Top"=w409:i16)  [unwired: 2 out]
        n174 = Unbundle(w414) -> ("Left"=w411:i16, "Top"=w410:i16)  [unwired: 2 out]
        n175 = Unbundle(w416) -> ("Left"=w408:i16, "Top"=w405:i16)  [unwired: 2 out]
        n176 = Not Equal?(x=w405, y=w407) -> (x != y?=w403:bool)
        n177 = Not Equal?(x=w409, y=w410) -> (x != y?=w401:bool)
        n178 = Not Equal?(x=w408, y=w406) -> (x != y?=w404:bool)
        n179 = Not Equal?(x=w412, y=w411) -> (x != y?=w402:bool)
        n180 = Compound Arithmetic op=OR(w404, w403, w402, w401) -> (w400:bool)
        n181 = case shown="True" w400 {
          tunnel: w424 -> [w435 w456]
          tunnel: w423 -> [w436 w455]
          tunnel: [w436 w443] -> w422
          tunnel: [w435 w441] -> w421
          tunnel: w416 -> [_ w440]
          tunnel: w415 -> [_ w439]
          tunnel: w414 -> [_ w438]
          tunnel: w413 -> [_ w437]
          frame False {
          }
          frame True {
            n182 = Subtract(x=w440, y=w437) -> (x-y=w453:T7)
            n183 = Subtract(x=w439, y=w438) -> (x-y=w446:T7)
            n184 = Unbundle(w453) -> ("Left"=w452:i16, "Top"=w451:i16)  [unwired: 2 out]
            n185 = Unbundle(w446) -> ("Left"=w447:i16, "Top"=w448:i16)  [unwired: 2 out]
            n186 = Bundle(cluster=w437, "Left"=w452, "Top"=w451, "Right"=w452, "Bottom"=w451) -> (w450:T7)
            n187 = Bundle(cluster=w438, "Left"=w447, "Top"=w448, "Right"=w447, "Bottom"=w448) -> (w449:T7)
            n188 = Subtract(x=w440, y=w450) -> (x-y=w454:T7)
            n189 = Subtract(x=w439, y=w449) -> (x-y=w445:T7)
            n190 = property class="VI"(reference=w456, error in=w455, "Front Panel.WinBounds"=w454, "BDWin.Bounds"=w445) -> (reference out=w442:refnum<vi>, error out=w444:errorcluster)
            n191 = invoke class="VI" method="Save.Instrument"(reference=w442, error in=w444) -> (reference out=w441:refnum<vi>, error out=w443:errorcluster)  [unwired: 4 in, 4 out]
          }
        }
        n192 = Close Reference(reference=w421, error in (no error)=w422) -> (error out=w431:errorcluster)
        n193 = call <vilib>:"Add State(s) to Queue__JKI_lib_State_Machine.vi"("State(s) in Front (\"\")"="UI: Post Action" ("State(s) in Front (\"\")"), "State(s) in (\"\")"=w428) -> ("States Out"=w429:string)  [unwired: 13 in]
        n194 = Not(x=w431) -> (.not. x?=w430:bool)
        n195 = Bundle By Name(cluster=w398, "Success"=w430) -> (w432:T4)
      }
      frame "Action: Open If Inline" {
        n196 = String To Path(string=w480) -> (path=w481:path)
        n197 = Unbundle By Name(w469) -> ("Root"=w470:path)
        n198 = Build Path(base path=w470, name or relative path=w481) -> (appended path=w472:path)
        n199 = Open VI Reference(vi path=w472, options=2) -> (vi reference=w465:refnum<vi>, error out=w471:errorcluster)  [unwired: 4 in]
        n200 = property class="VI"(reference=w465, error in=w471) -> (reference out=w464:refnum<vi>, error out=w466:errorcluster, "ExecInlining"=w463:bool)
        n201 = case shown="True" w463 {
          tunnel: [w483 w487] -> w468
          tunnel: [w482 w486] -> w467
          tunnel: w466 -> [w483 w485]
          tunnel: w464 -> [w482 w484]
          frame False {
          }
          frame True {
            n202 = invoke class="VI" method="FP.Open"(reference=w484, error in=w485) -> (reference out=w486:refnum<vi>, error out=w487:errorcluster)  [unwired: 3 in, 3 out]
          }
        }
        n203 = Close Reference(reference=w467, error in (no error)=w468) -> (error out=w478:errorcluster)
        n204 = call <vilib>:"Add State(s) to Queue__JKI_lib_State_Machine.vi"("State(s) in Front (\"\")"="UI: Post Action" ("State(s) in Front (\"\")"), "State(s) in (\"\")"=w475) -> ("States Out"=w476:string)  [unwired: 13 in]
        n205 = Not(x=w478) -> (.not. x?=w477:bool)
        n206 = Bundle By Name(cluster=w469, "Success"=w477) -> (w479:T4)
      }
      frame "Action: Update VI Title" {
        w512 = "(CSM)" ("string")
        n207 = String To Path(string=w502) -> (path=w503:path)
        n208 = Unbundle By Name(w495) -> ("Root"=w496:path)
        n209 = Build Path(base path=w496, name or relative path=w503) -> (appended path=w501:path)
        n210 = Strip Path(path=w501) -> (name=w509:string)  [unwired: 1 out]
        n211 = Open VI Reference(vi path=w501, options=2) -> (vi reference=w518:refnum<vi>, error out=w520:errorcluster)  [unwired: 4 in]
        n212 = Match Pattern(string=w509, regular expression=".vi[m]?$") -> (before substring=w514:string)  [unwired: 1 in, 3 out]
        n213 = property class="VI"(reference=w518, error in=w520) -> (reference out=w517:refnum<vi>, error out=w519:errorcluster, "Front Panel.Title"=w493:string)
        n214 = Match Pattern(string=w493, regular expression=w512) -> (offset past match=w515:i32)  [unwired: 1 in, 3 out]
        n215 = Greater Or Equal To 0?(x=w515) -> ()  [unwired: 1 out]
        n216 = Match Pattern(string=w493, regular expression="[.]+$") -> (offset past match=w489:i32)  [unwired: 1 in, 3 out]
        n217 = Select(t=w493, s=FALSE, f=w514) -> (s? t:f=w513:string)
        n218 = Search and Replace String(replace all?=TRUE ("replace all? (F)"), input string=w513, search string=w512) -> (result string=w510:string)  [unwired: 5 in, 3 out]
        n219 = call <vilib>:"Trim Whitespace.vi"("string"=w510) -> ("trimmed string"=w508:string)  [unwired: 1 in]
        n220 = Concatenate Strings(w508, " (CSM)" ("string")) -> (w507:string)
        n221 = Less Than 0?(x=w489) -> (x < 0?=w488:bool)
        n222 = Not Equal?(x=w493, y=w507) -> (x != y?=w491:bool)
        n223 = And(x=w491, y=w488) -> (x .and. y?=w490:bool)
        n224 = case shown="True" w490 {
          tunnel: [w525 w532] -> w523
          tunnel: [w524 w531] -> w522
          tunnel: w519 -> [w525 w530]
          tunnel: w517 -> [w524 w529]
          tunnel: w507 -> [_ w527]
          frame False {
          }
          frame True {
            n225 = property class="VI"(reference=w529, error in=w530, "Front Panel.Title"=w527) -> (reference out=w528:refnum<vi>, error out=w526:errorcluster)
            n226 = invoke class="VI" method="Save.Instrument"(reference=w528, error in=w526) -> (reference out=w531:refnum<vi>, error out=w532:errorcluster)  [unwired: 4 in, 4 out]
          }
        }
        n227 = Close Reference(reference=w522, error in (no error)=w523) -> (error out=w498:errorcluster)
        n228 = call <vilib>:"Add State(s) to Queue__JKI_lib_State_Machine.vi"("State(s) in Front (\"\")"="UI: Post Action" ("State(s) in Front (\"\")"), "State(s) in (\"\")"=w505) -> ("States Out"=w506:string)  [unwired: 13 in]
        n229 = Bundle("name"=w509, "error out"=w498) -> ()  [unwired: 1 in, 1 out]
        n230 = Not(x=w498) -> (.not. x?=w497:bool)
        n231 = Bundle By Name(cluster=w495, "Success"=w497) -> (w499:T4)
      }
      frame "Action: Set Debugging" {
        n232 = String To Path(string=w544) -> (path=w545:path)
        n233 = Unbundle By Name(w537) -> ("Root"=w538:path)
        n234 = Build Path(base path=w538, name or relative path=w545) -> (appended path=w543:path)
        n235 = Open VI Reference(vi path=w543, options=2) -> (vi reference=w550:refnum<vi>, error out=w552:errorcluster)  [unwired: 4 in]
        n236 = property class="VI"(reference=w550, error in=w552) -> (reference out=w549:refnum<vi>, error out=w551:errorcluster, "Exec.AllowDebug"=w536:bool)
        n237 = Not Equal?(x="Option", y=w536) -> (x != y?=w535:bool)
        n238 = case shown="True" w535 {
          tunnel: [w556 w564] -> w554
          tunnel: [w555 w563] -> w553
          tunnel: w551 -> [w556 w562]
          tunnel: w549 -> [w555 w561]
          tunnel: "Option" -> [_ w558]
          tunnel: "Enum" -> [_ w557]
          frame False {
          }
          frame True {
            n239 = case shown="\"AutoErrorHandling\"" w557 {
              tunnel: w562 -> [w569 w574]
              tunnel: w561 -> [w568 w573]
              tunnel: [w567 w572] -> w560
              tunnel: [w566 w571] -> w559
              tunnel: w558 -> [w565 w570]
              frame "Debugging", Default {
                n240 = property class="VI"(reference=w568, error in=w569, "Exec.AllowDebug"=w565) -> (reference out=w567:refnum<vi>, error out=w566:errorcluster)
              }
              frame "AutoErrorHandling" {
                n241 = property class="VI"(reference=w573, error in=w574, "Def Err Handling"=w570) -> (reference out=w572:refnum<vi>, error out=w571:errorcluster)
              }
            }
            n242 = invoke class="VI" method="Save.Instrument"(reference=w560, error in=w559) -> (reference out=w563:refnum<vi>, error out=w564:errorcluster)  [unwired: 4 in, 4 out]
          }
        }
        n243 = Close Reference(reference=w553, error in (no error)=w554) -> (error out=w540:errorcluster)
        n244 = call <vilib>:"Add State(s) to Queue__JKI_lib_State_Machine.vi"("State(s) in Front (\"\")"="UI: Post Action" ("State(s) in Front (\"\")"), "State(s) in (\"\")"=w547) -> ("States Out"=w548:string)  [unwired: 13 in]
        n245 = Not(x=w540) -> (.not. x?=w539:bool)
        n246 = Bundle By Name(cluster=w537, "Success"=w539) -> (w541:T4)
      }
      frame "Action: Update Connect Panel Doc" {
        n247 = Unbundle By Name(w577) -> ("Root"=w578:path)
        n248 = String To Path(string=w581) -> (path=w582:path)
        n249 = Build Path(base path=w578, name or relative path=w582) -> (appended path=w576:path)
        n250 = call "Update Connect Panel Doc.vi"("vi path"=w576) -> ("error out"=w575:errorcluster)  [unwired: 9 in, 1 out]
        n251 = call <vilib>:"Add State(s) to Queue__JKI_lib_State_Machine.vi"("State(s) in Front (\"\")"="UI: Post Action" ("State(s) in Front (\"\")"), "State(s) in (\"\")"=w584) -> ("States Out"=w585:string)  [unwired: 13 in]
        n252 = Not(x=w575) -> (.not. x?=w579:bool)
        n253 = Bundle By Name(cluster=w577, "Success"=w579) -> (w580:T4)
      }
    }
  }
